vi "Untitled 1.vi"() -> ()   [LabVIEW 2019]
panel:
  out "data out 2":string
  out "error out":errorcluster
  out "data out":string
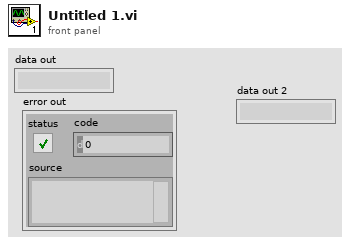
[diagram p1: front panel]
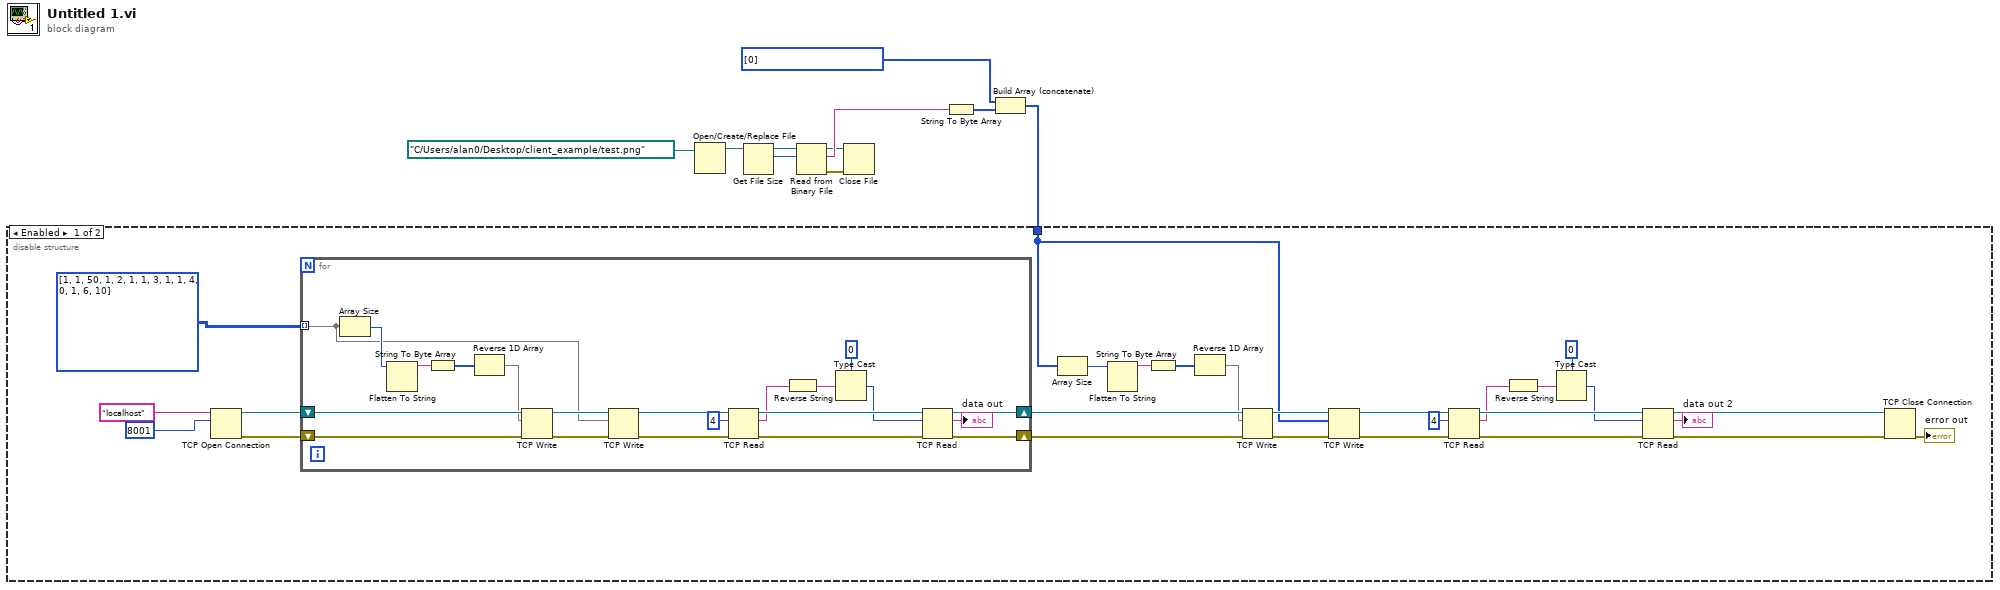
[diagram p0: block diagram]
diagram:
  n1 = Open/Create/Replace File(file path (use dialog)=path "C:/Users/alan0/Desktop/client_example/test.png" ("path to PNG file")) -> (refnum out=w6:refnum<file>)  [unwired: 5 in, 2 out]
  n2 = Get File Size(file=w6) -> (refnum out=w5:refnum<file>, size (in bytes)=w2:i64)  [unwired: 1 in, 1 out]
  n3 = Read from Binary File(10:w2, 11:w5) -> (0:w4:errorcluster, 2:w8:string, 3:w3:refnum<file>)  [unwired: 4 in, 1 out]
  n4 = Close File(refnum=w3, error in=w4) -> ()  [unwired: 2 out]
  n5 = String To Byte Array(string=w8) -> (unsigned byte array=w10:u8[])
  n6 = Build Array (concatenate)(u8[] [0], w10) -> (w1:u8[])
  n7 = disable-structure shown="Enabled" {
    disable-tunnel: w1 -> [w11 _]
    frame Enabled {
      n8 = TCP Open Connection(address="localhost", remote port or service name=u16 8001) -> (connection ID=w35:refnum<k5>, error out=w34:errorcluster)  [unwired: 3 in]
      n9 = for {
        tunnel: u8[][] [[1, 1, 50], [1, 2, 1], [1, 3, 1], [1, 4, 0], [1, 6, 10]] -> [w38] mode=indexing
        shift-right: [w46] -> w32
        shift-left: w35 -> [w58]
        shift-right: [w45] -> w31
        shift-left: w34 -> [w57]
        n10 = Array Size(array=w38) -> (size(s)=w54:i32)
        n11 = Flatten To String(anything=w54) -> (data string=w56:string)  [unwired: 3 in, 2 out]
        n12 = String To Byte Array(string=w56) -> (unsigned byte array=w55:u8[])
        n13 = Reverse 1D Array(array=w55) -> (reversed array=w53:u8[])
        n14 = TCP Write(connection ID=w58, data in=w53, error in (no error)=w57) -> (connection ID out=w52:refnum<k5>, error out=w51:errorcluster)  [unwired: 1 in, 1 out]
        n15 = TCP Write(connection ID=w52, data in=w38, error in (no error)=w51) -> (connection ID out=w50:refnum<k5>, error out=w49:errorcluster)  [unwired: 1 in, 1 out]
        n16 = TCP Read(connection ID=w50, bytes to read=4, error in (no error)=w49) -> (connection ID out=w48:refnum<k5>, data out=w43:string, error out=w47:errorcluster)  [unwired: 2 in]
        n17 = Reverse String(1:w43) -> (0:w39:string)
        n18 = Type Cast(type=0 ("bytes to read"), x=w39) -> (*(type *) &x=w41:i32)
        n19 = TCP Read(connection ID=w48, bytes to read=w41, error in (no error)=w47) -> (connection ID out=w46:refnum<k5>, data out=→"data out":string, error out=w45:errorcluster)  [unwired: 2 in]
      }
      n20 = Array Size(array=w11) -> (size(s)=w25:i32)
      n21 = Flatten To String(anything=w25) -> (data string=w27:string)  [unwired: 3 in, 2 out]
      n22 = String To Byte Array(string=w27) -> (unsigned byte array=w26:u8[])
      n23 = Reverse 1D Array(array=w26) -> (reversed array=w24:u8[])
      n24 = TCP Write(connection ID=w32, data in=w24, error in (no error)=w31) -> (connection ID out=w23:refnum<k5>, error out=w22:errorcluster)  [unwired: 1 in, 1 out]
      n25 = TCP Write(connection ID=w23, data in=w11, error in (no error)=w22) -> (connection ID out=w21:refnum<k5>, error out=w20:errorcluster)  [unwired: 1 in, 1 out]
      n26 = TCP Read(connection ID=w21, bytes to read=4, error in (no error)=w20) -> (connection ID out=w19:refnum<k5>, data out=w16:string, error out=w18:errorcluster)  [unwired: 2 in]
      n27 = Reverse String(1:w16) -> (0:w12:string)
      n28 = Type Cast(type=0 ("bytes to read"), x=w12) -> (*(type *) &x=w14:i32)
      n29 = TCP Read(connection ID=w19, bytes to read=w14, error in (no error)=w18) -> (connection ID out=w29:refnum<k5>, data out=→"data out 2":string, error out=w30:errorcluster)  [unwired: 2 in]
      n30 = TCP Close Connection(connection ID=w29, error in (no error)=w30) -> (error out=→"error out":errorcluster)  [unwired: 1 in, 1 out]
    }
    frame Disabled {
    }
  }
